vi "MoveThetaAbs.vi"(8 "Theta":dbl, 10 "error out 2":errorcluster, 11 "connection ID":refnum<k5>) -> (0 "ThetaOut (rad)":dbl, 2 "error out":errorcluster, 3 "connection ID 2":refnum<k5>)   [LabVIEW 2018]
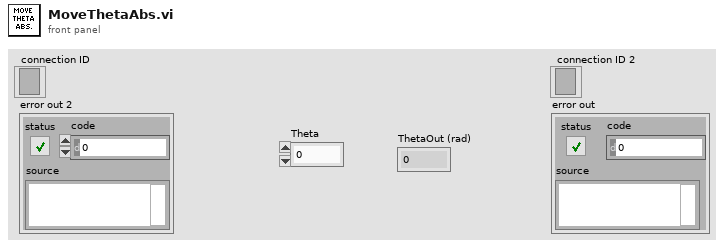
[diagram p1: front panel]
types:
  T1 = enum16{"Standard", "Buffered", "CRLF", "Immediate"}
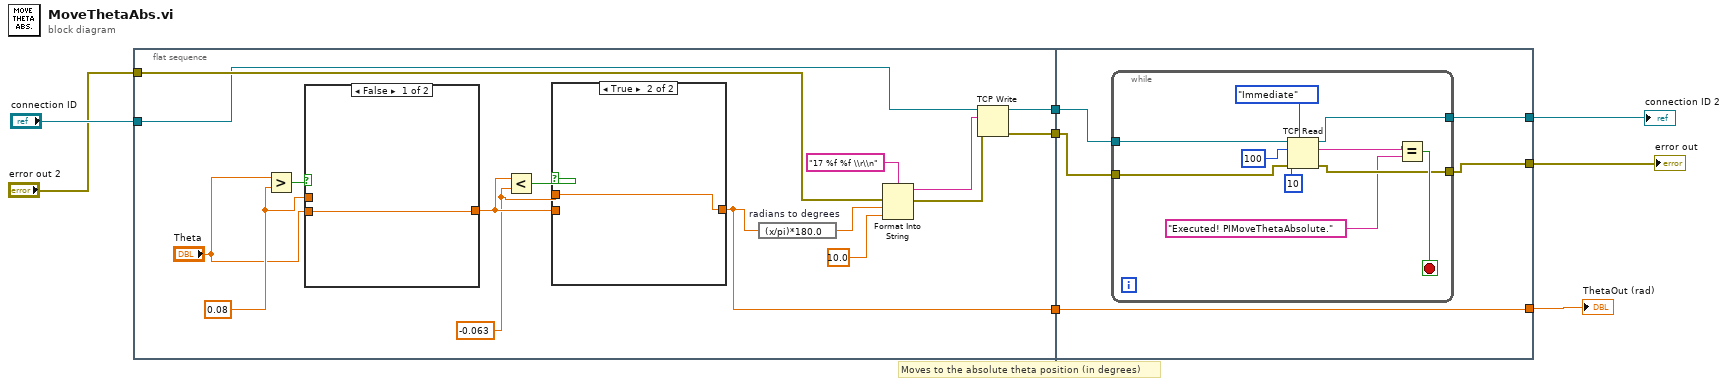
[diagram p0: block diagram]
diagram:
  # "Moves to the absolute theta position (in degrees)"
  n1 = flat-sequence {
    tunnel: [w22] -> w8
    tunnel: [w21] -> w7
    tunnel: "error out 2" -> [w14]
    tunnel: "connection ID" -> [w13]
    tunnel: [w10] -> w2
    tunnel: w8 -> [w32]
    tunnel: w7 -> [w33]
    tunnel: [w31] -> w4
    tunnel: [w30] -> w3
    tunnel: [w29] -> w1
    tunnel: w2 -> [w29]
    frame #0 {
      w16 = 0.08 ("y")
      w15 = -0.063 ("y")
      n2 = Greater?(x="Theta", y=w16) -> (0:w18:bool)
      n3 = case shown="False" w18 {
        tunnel: "Theta" -> [w27 _]
        tunnel: [w27 w28] -> w17
        tunnel: w16 -> [_ w28]
        frame False {
        }
        frame True {
        }
      }
      n4 = Less?(x=w17, y=w15) -> (x < y?=w20:bool)
      n5 = case shown="True" w20 {
        tunnel: [w25 w26] -> w10
        tunnel: w17 -> [w25 _]
        tunnel: w15 -> [_ w26]
        frame False {
        }
        frame True {
        }
      }
      n6 = expression code="(x/pi)*180.0" "radians to degrees"(w10) -> (w9:dbl)
      n7 = Format Into String(format string="17 %f %f \\r\\n", error in=w14, w9, 10.0 ("input 3")) -> (resulting string=w23:string, error out=w24:errorcluster)  [unwired: 1 in]
      n8 = TCP Write(connection ID=w13, data in=w23, error in (no error)=w24) -> (connection ID out=w22:refnum<k5>, error out=w21:errorcluster)  [unwired: 1 in, 1 out]
    }
    frame #1 {
      n9 = while {
        tunnel: w33 -> [w41]
        tunnel: [w37] -> w30
        tunnel: [w36] -> w31
        tunnel: w32 -> [w34]
        stop <- w38 stop-if-true
        n10 = TCP Read(connection ID=w34, bytes to read=100, error in (no error)=w41, 7:T1."Immediate" ("mode (standard)"), 9:10 ("timeout ms (25000)")) -> (connection ID out=w36:refnum<k5>, data out=w39:string, error out=w37:errorcluster)
        n11 = Equal?(x=w39, y="Executed! PIMoveThetaAbsolute.") -> (x = y?=w38:bool)
      }
    }
  }
  "connection ID 2" <- w4
  "error out" <- w3
  "ThetaOut (rad)" <- w1
